vi "uMsg Get Latency.vi"(8 "error in (no error)":errorcluster, 11 "uMsg in":refnum<class "uMsg.lvclass">) -> (0 "error out":errorcluster, 2 "Latency (ms)":u32, 3 "uMsg out":refnum<class "uMsg.lvclass">)   [LabVIEW 2021, in "uFramework.lvlib" / "uMsg.lvclass"]
doc: "Return the time that has elapsed since the messsage has updates its timestamp"
uses:
  uMsg.lvclass
  uMsg.lvclass/uMsg.ctl
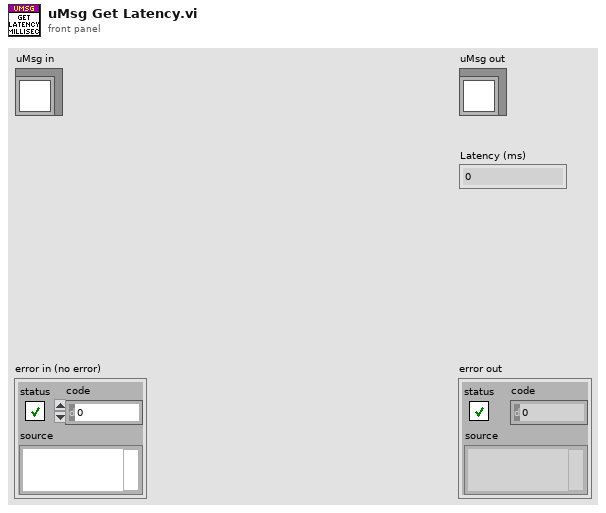
[diagram p1: front panel]
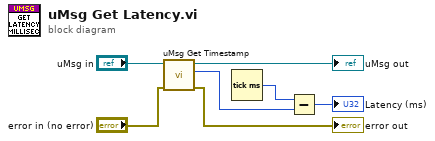
[diagram p0: block diagram]
diagram:
  n1 = call "uMsg Get Timestamp.vi"("error in (no error)"="error in (no error)", "uMsg in"="uMsg in") -> ("error out"=→"error out":errorcluster, "Tick Count"=w5:u32, "uMsg out"=→"uMsg out":refnum<class "uMsg.lvclass">)  [unwired: 7 in]
  n2 = Tick Count (ms)() -> (millisecond timer value=w4:u32)
  n3 = Subtract(x=w4, y=w5) -> (x-y=→"Latency (ms)":u32)
